vi "TTA_EXA_GetACPR.vi"(0 "VISA resource In":refnum<visa-resource-name>, 5 "Frequency (MHz)":dbl, 11 "error in":errorcluster) -> (4 "VISA resource Out":refnum<visa-resource-name>, 6 "ACP Values":dbl[](array[numeric]), 8 "ACP Sorted":dbl[](array[numeric]), 15 "error out":errorcluster)   [LabVIEW 2016]
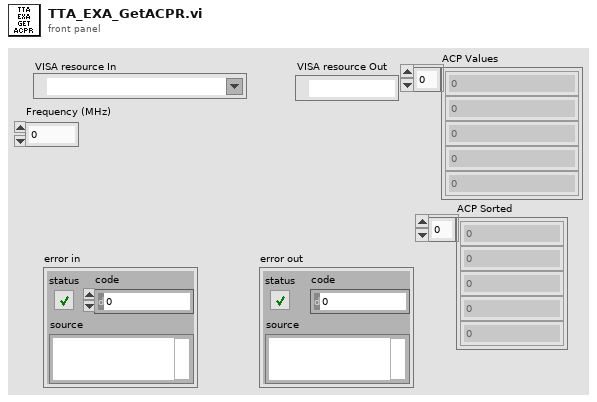
[diagram p1: front panel]
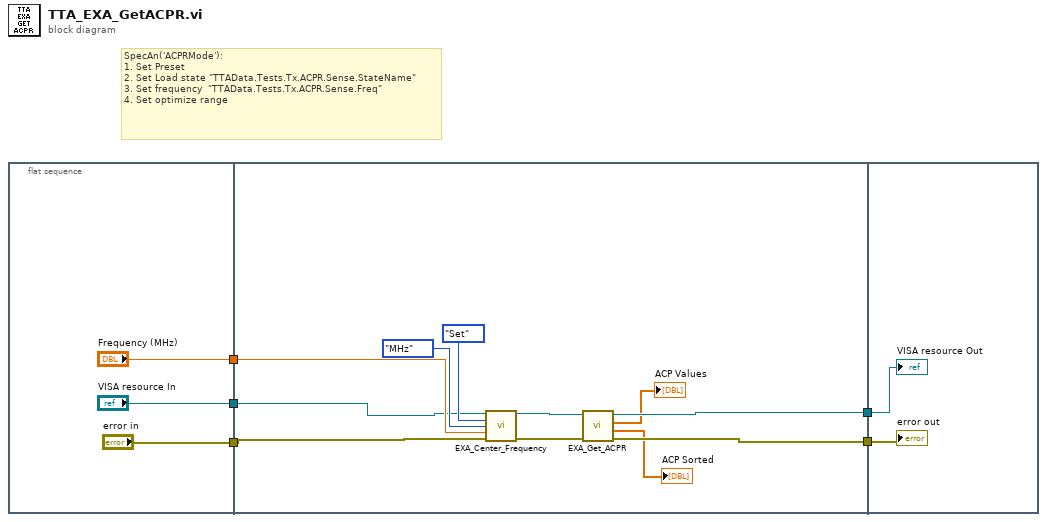
[diagram p0: block diagram]
diagram:
  # "SpecAn('ACPRMode'):\n1. Set Preset\n2. Set Load state \"TTAData.Tests.Tx.ACPR.Sense.StateName\"\n3. Set frequency  \"TTAData.Tests.Tx.ACPR.Sense.Freq\"\n4. Set optimize range"
  n1 = flat-sequence {
    tunnel: ["error in"] -> w5
    tunnel: ["VISA resource In"] -> w4
    tunnel: ["Frequency (MHz)"] -> w3
    tunnel: w5 -> [w15]
    tunnel: w4 -> [w16]
    tunnel: w3 -> [w19]
    tunnel: [w12] -> w2
    tunnel: [w11] -> w1
    tunnel: w2 -> [w21]
    tunnel: w1 -> [w20]
    frame #0 {
    }
    frame #1 {
      n2 = call "EXA_Center_Frequency.vi"("VISA resource name"=w16, "Mode"=enum16{"Set", "Get"}."Set", "Units"=enum16{"Hz", "kHz", "MHz", "GHz"}."MHz", "Frequency"=w19, "error in"=w15) -> ("VISA resource name"=w13:refnum<visa-resource-name>, "error out"=w14:errorcluster)  [unwired: 8 in, 1 out]
      n3 = call "EXA_Get_ACPR.vi"("error in"=w14, "VISA resource name"=w13) -> ("error out"=w11:errorcluster, "ACP Sorted"=→"ACP Sorted":dbl[], "ACP Values"=→"ACP Values":dbl[], "VISA resource name"=w12:refnum<visa-resource-name>)  [unwired: 6 in]
    }
    frame #2 {
      "VISA resource Out" <- w21
      "error out" <- w20
    }
  }
